vi "Check Corruption.vi"(11 "input string":string) -> (2 "Boolean":bool, 3 "Array":bool[](array[boolean]))   [LabVIEW 2019, in "Day 10.lvlib"]
uses:
  Day 10.lvlib
panel:
  out "< >":i32
  out "{ }":i32
  out "[ ]":i32
  out "( )":i32
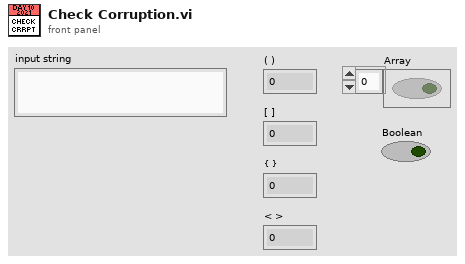
[diagram p1: front panel]
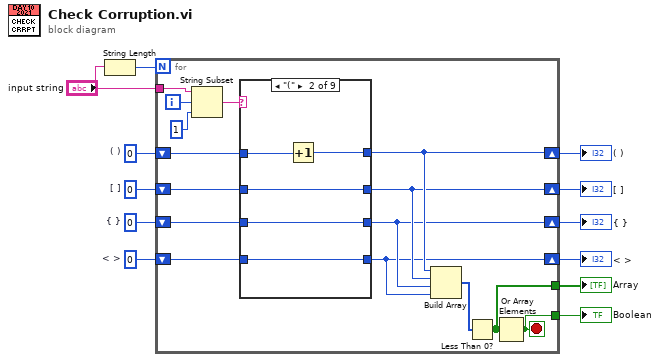
[diagram p0: block diagram]
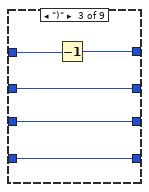
[diagram p3: hidden frame]
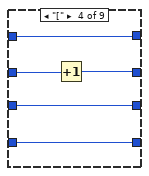
[diagram p4: hidden frame]
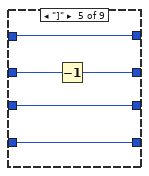
[diagram p5: hidden frame]
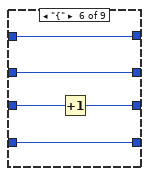
[diagram p6: hidden frame]
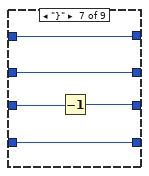
[diagram p7: hidden frame]
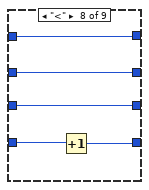
[diagram p8: hidden frame]
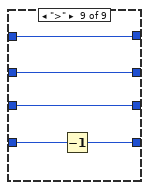
[diagram p9: hidden frame]
diagram:
  w10 = 0  # < >
  w9 = 0  # { }
  w8 = 0  # [ ]
  w7 = 0  # ( )
  n1 = String Length(string="input string") -> (length=w6:i32)
  n2 = for {
    N: w6 -> [_]
    tunnel: "input string" -> [w27]
    shift-right: [w19] -> w4
    shift-left: w7 -> [w23]
    shift-right: [w18] -> w3
    shift-left: w8 -> [w22]
    shift-right: [w17] -> w2
    shift-left: w9 -> [w21]
    shift-right: [w16] -> w1
    shift-left: w10 -> [w20]
    tunnel: [w15] -> w12
    tunnel: [w13] -> w11
    i -> [w26]
    stop <- w15 stop-if-true
    n3 = String Subset(string=w27, offset (0)=w26, length (rest)=1 ("length (rest)")) -> (substring=w24:string)
    n4 = case shown="\"(\"" w24 {
      tunnel: w23 -> [w31 w36 w41 w44 w49 w54 w61 w66 w71]
      tunnel: [w31 w35 w40 w44 w49 w54 w61 w66 w71] -> w19
      tunnel: [w30 w34 w39 w42 w47 w56 w60 w65 w70] -> w18
      tunnel: w22 -> [w30 w34 w39 w43 w48 w56 w60 w65 w70]
      tunnel: [w29 w33 w38 w46 w51 w52 w57 w64 w69] -> w17
      tunnel: w21 -> [w29 w33 w38 w46 w51 w53 w58 w64 w69]
      tunnel: [w28 w32 w37 w45 w50 w55 w59 w62 w67] -> w16
      tunnel: w20 -> [w28 w32 w37 w45 w50 w55 w59 w63 w68]
      frame Default {
      }
      frame "(" {
        n5 = Increment(x=w36) -> (x+1=w35:i32)
      }
      frame ")" {
        n6 = Decrement(x=w41) -> (x-1=w40:i32)
      }
      frame "[" {
        n7 = Increment(x=w43) -> (x+1=w42:i32)
      }
      frame "]" {
        n8 = Decrement(x=w48) -> (x-1=w47:i32)
      }
      frame "{" {
        n9 = Increment(x=w53) -> (x+1=w52:i32)
      }
      frame "}" {
        n10 = Decrement(x=w58) -> (x-1=w57:i32)
      }
      frame "<" {
        n11 = Increment(x=w63) -> (x+1=w62:i32)
      }
      frame ">" {
        n12 = Decrement(x=w68) -> (x-1=w67:i32)
      }
    }
    n13 = Build Array(w19, w18, w17, w16) -> (w14:i32[])
    n14 = Less Than 0?(x=w14) -> (x < 0?=w13:bool[])
    n15 = Or Array Elements(Boolean array=w13) -> (logical OR=w15:bool)
  }
  "Boolean" <- w12
  "Array" <- w11
  "( )" <- w4
  "[ ]" <- w3
  "{ }" <- w2
  "< >" <- w1
